vi "SWERVE_DRIVE_GET_MAX.vi"() -> (1 "Max Rotational Vel (Rad/Sec)":dbl, 3 "Max Wheel Vel (Meter/Sec)":dbl)   [LabVIEW 2023]
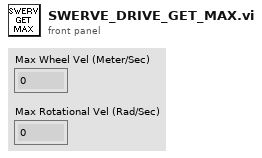
[diagram p1: front panel]
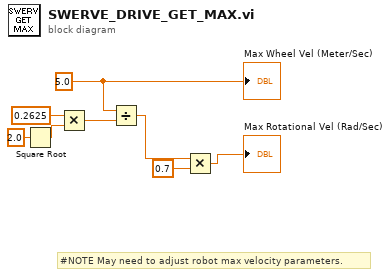
[diagram p0: block diagram]
diagram:
  w4 = 5.0
  # "#NOTE May need to adjust robot max velocity parameters."
  n1 = Square Root(x=2.0) -> (sqrt(x)=w7:dbl)
  n2 = Multiply(x=0.2625 ("X"), y=w7) -> (x*y=w5:dbl)
  n3 = Divide(x=w4, y=w5) -> (x/y=w3:dbl)
  n4 = Multiply(x=w3, y=0.7) -> (x*y=→"Max Rotational Vel (Rad/Sec)":dbl)
  "Max Wheel Vel (Meter/Sec)" <- w4
